vi "Read.vi"(8 "error in (no error)":errorcluster, 11 "Const_WFM in":refnum<class "Const_WFM.lvclass">) -> (0 "error out":errorcluster, 2 "Waveform":waveform(dbl), 3 "Const_WFM out":refnum<class "Const_WFM.lvclass">)   [LabVIEW 2021, in "Const_WFM.lvclass"]
uses:
  Const_WFM.lvclass
  Const_WFM.lvclass/Const_WFM.ctl
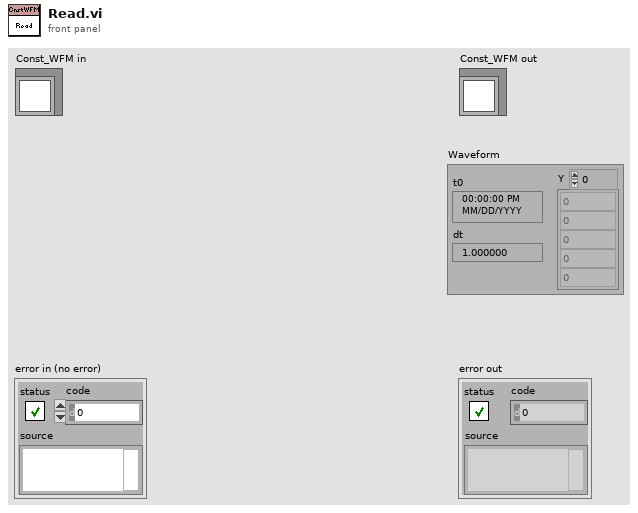
[diagram p1: front panel]
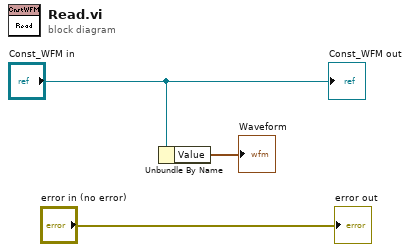
[diagram p0: block diagram]
diagram:
  n1 = Unbundle By Name("Const_WFM in") -> ("Value"=→"Waveform":waveform(dbl))
  "error out" <- "error in (no error)"
  "Const_WFM out" <- "Const_WFM in"
